vi "Get Shooter Angle.vi"() -> (3 "Current Angle":dbl)   [LabVIEW 2015]
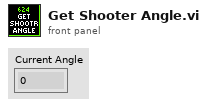
[diagram p1: front panel]
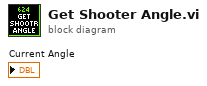
[diagram p0: block diagram]
diagram:
